vi "Message generator.vi"(8 "error in":errorcluster, 10 "Account info":string, 11 "Message":T2) -> (0 "error out":errorcluster, 1 "ATM Message":string, 2 "Left Menu":T1, 3 "Right Menu":T1)   [LabVIEW 2015]
doc: "Generate messages to dispaly on ATM messages Control, and Right/Left menu."
uses:
  Controls/Message.ctl
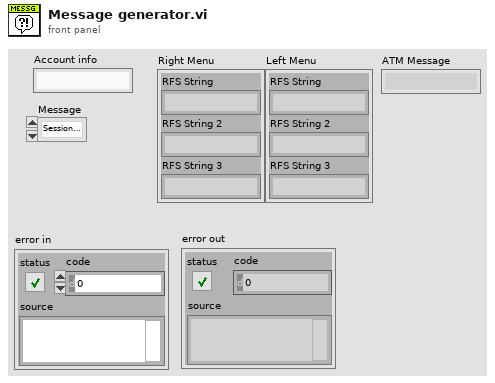
[diagram p1: front panel]
types:
  T1 = cluster{"RFS String":string, "RFS String 2":string, "RFS String 3":string}
  T2 = typedef "Message.ctl" = enum16{"Session Terminate ", "Account Verification Failed", "Main Menu ", "Balance Inquiry", "Withdrawal Failed", "Withdrawal Complete", "Withdrawal", "Deposit Complete", "Deposit ", "Welcome "}
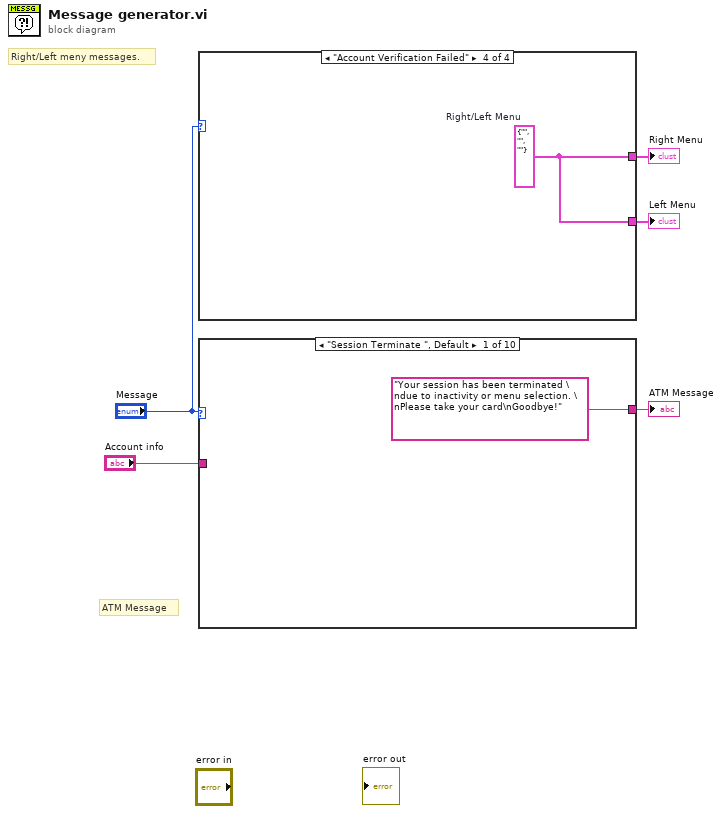
[diagram p0: block diagram]
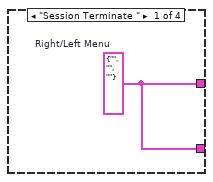
[diagram p2: hidden frame]
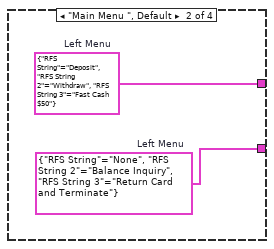
[diagram p3: hidden frame]
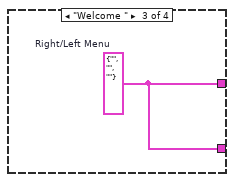
[diagram p4: hidden frame]
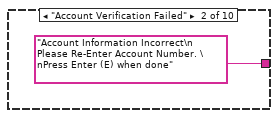
[diagram p5: hidden frame]
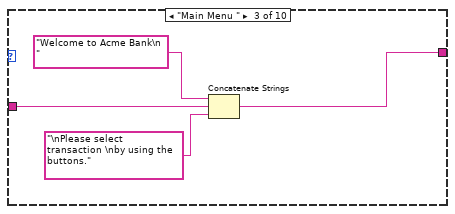
[diagram p6: hidden frame]
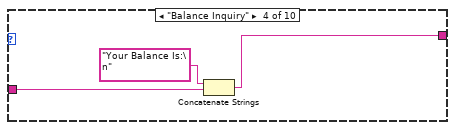
[diagram p7: hidden frame]
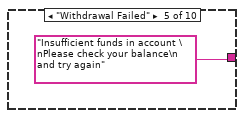
[diagram p8: hidden frame]
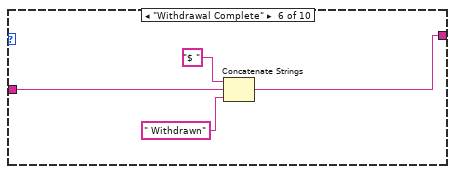
[diagram p9: hidden frame]
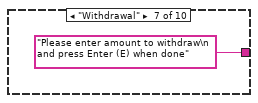
[diagram p10: hidden frame]
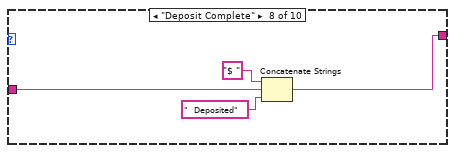
[diagram p11: hidden frame]
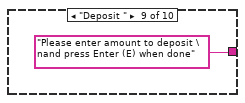
[diagram p12: hidden frame]
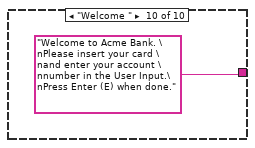
[diagram p13: hidden frame]
diagram:
  # "Right/Left meny messages."
  # "ATM Message"
  n1 = case shown="\"Account Verification Failed\"" "Message" {
    tunnel: [w6 w7 w9 w10] -> w4
    tunnel: [w6 w8 w9 w10] -> w3
    frame "Session Terminate " {
      w6 = T1 {"RFS String"="", "RFS String 2"="", "RFS String 3"=""}  # Right/Left Menu
    }
    frame "Main Menu ", Default {
      w7 = T1 {"RFS String"="Deposit", "RFS String 2"="Withdraw", "RFS String 3"="Fast Cash $50"}  # Left Menu
      w8 = T1 {"RFS String"="None", "RFS String 2"="Balance Inquiry", "RFS String 3"="Return Card and Terminate"}  # Left Menu
    }
    frame "Welcome " {
      w9 = T1 {"RFS String"="", "RFS String 2"="", "RFS String 3"=""}  # Right/Left Menu
    }
    frame "Account Verification Failed" {
      w10 = T1 {"RFS String"="", "RFS String 2"="", "RFS String 3"=""}  # Right/Left Menu
    }
  }
  "Right Menu" <- w4
  "Left Menu" <- w3
  n2 = case shown="\"Session Terminate \", Default" "Message" {
    tunnel: ["Your session has been terminated \ndue to inactivity or menu selection. \nPlease take your card\nGoodbye!" "Account Information Incorrect\n Please Re-Enter Account Number. \nPress Enter (E) when done" w13 w17 "Insufficient funds in account \nPlease check your balance\n and try again" ("string") w21 "Please enter amount to withdraw\n and press Enter (E) when done" ("string") w26 "Please enter amount to deposit \nand press Enter (E) when done" "Welcome to Acme Bank. \nPlease insert your card \nand enter your account \nnumber in the User Input.\nPress Enter (E) when done."] -> w2
    tunnel: "Account info" -> [_ _ w15 w18 _ w22 _ w28 _ _]
    frame "Session Terminate ", Default {
    }
    frame "Account Verification Failed" {
    }
    frame "Main Menu " {
      n3 = Concatenate Strings("Welcome to Acme Bank\n ", w15, "\nPlease select transaction \nby using the buttons." ("string")) -> (w13:string)
    }
    frame "Balance Inquiry" {
      n4 = Concatenate Strings("Your Balance Is:\n" ("string"), w18) -> (w17:string)
    }
    frame "Withdrawal Failed" {
    }
    frame "Withdrawal Complete" {
      n5 = Concatenate Strings("$ " ("string"), w22, " Withdrawn" ("string")) -> (w21:string)
    }
    frame "Withdrawal" {
    }
    frame "Deposit Complete" {
      n6 = Concatenate Strings("$ " ("string"), w28, "  Deposited" ("string")) -> (w26:string)
    }
    frame "Deposit " {
    }
    frame "Welcome " {
    }
  }
  "ATM Message" <- w2
